vi "1-Main Image segmentation.vi"() -> ()   [LabVIEW 2015]
uses:
  <vilib>/Utility/file.llb/Read Delimited Spreadsheet (string).vi
  Dll/HyperImageBinarization.dll
panel:
  out "Image":T1(plugin-control)
  in  "secondOTSUMultiple":dbl
  in  "firstOTSUMultiple":dbl=0.94
  out "Current process of inter cycles":i32
  out "Number of inter cycles":i32
  out "Current process of external cycles":i32
  out "Number of external cycles":i32
  in  "divisor":i32=131
  in  "dividend":i32=109
  out "Current binary file path":path
  out "Files under current path":string[](array[string])
  out "lineNumbers":i32=340
  in  "waveSamples":i32=1004
  in  "waveNumbers":i32=250
  out "path":path
  in  "Binary path":path=path "I:/2017 Maize-Hyper-Program/2017 Maize Test sample/path.txt"
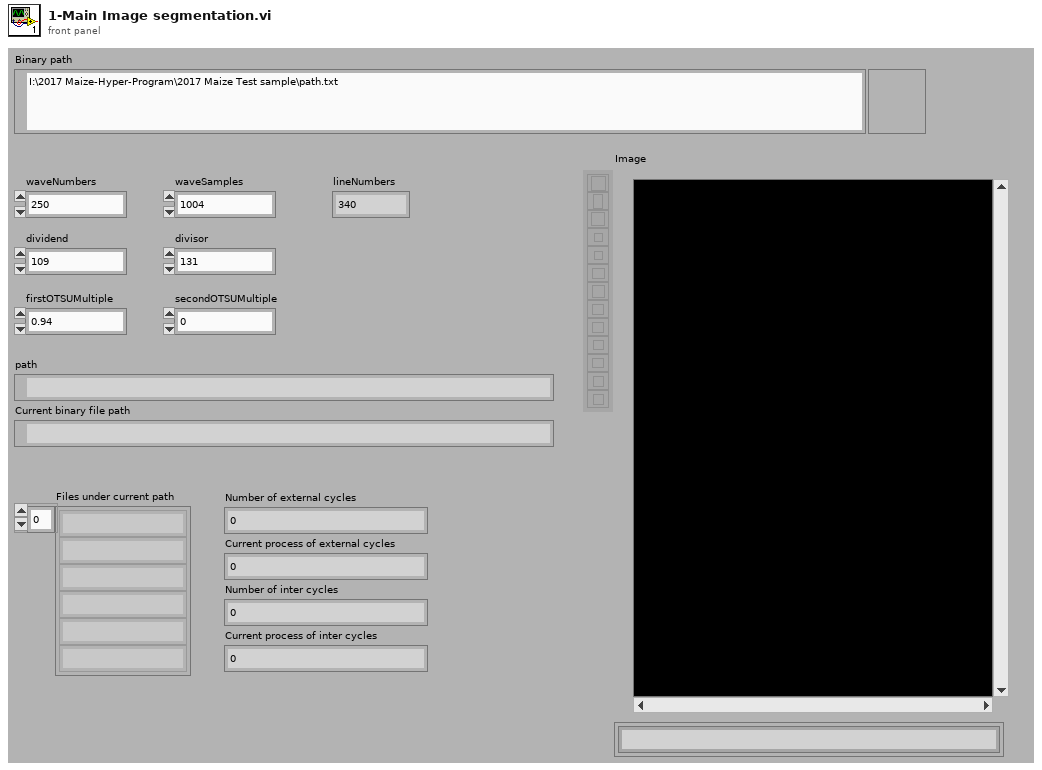
[diagram p1: front panel]
types:
  T1 = typedef "IMAQ Image.ctl" = refnum<image>
  T2 = typedef "Image Type" = u32
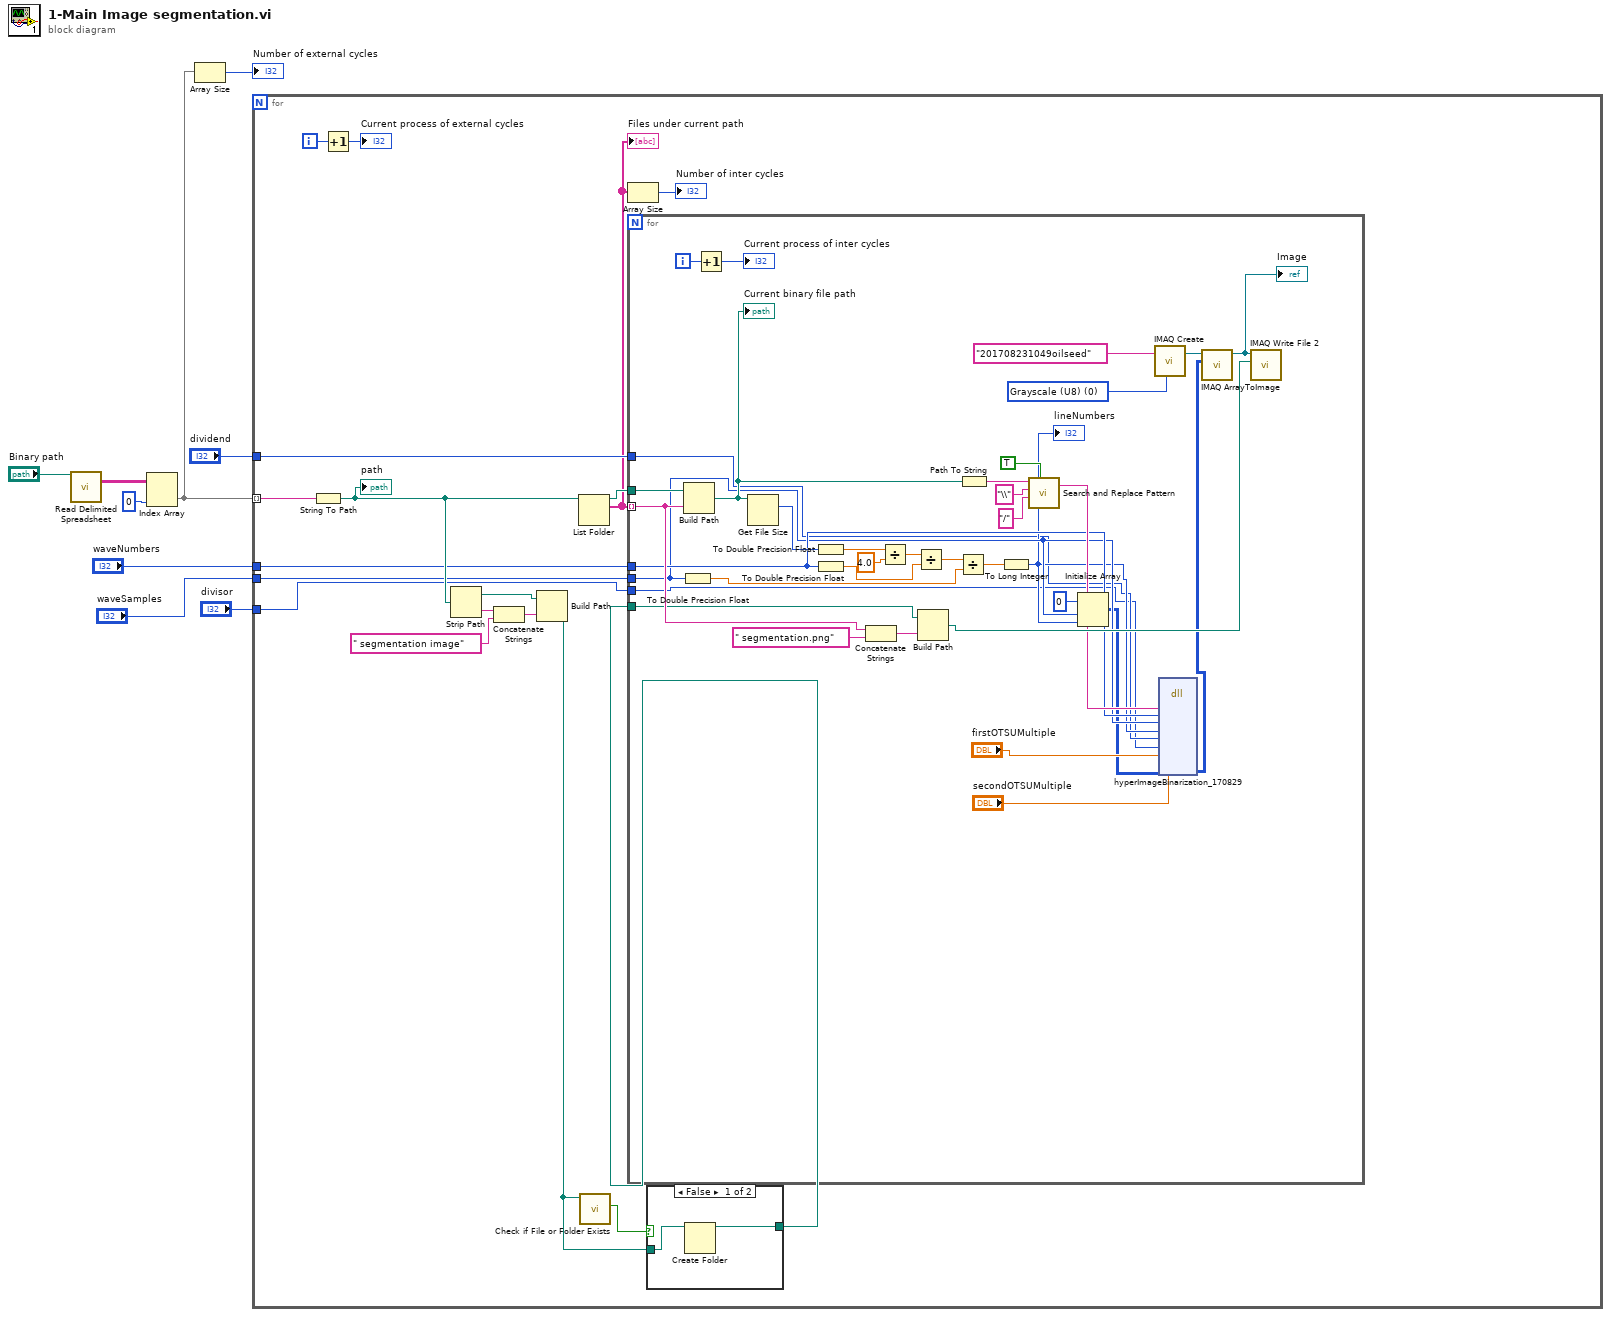
[diagram p0: block diagram]
diagram:
  n1 = call-poly <vilib>:"Read Delimited Spreadsheet.vi"("file path (dialog if empty)"="Binary path") -> ("all rows"=w5:string[][])  [unwired: 9 in, 5 out]
  n2 = Index Array(array=w5, index (col)=0 ("disabled index (col)")) -> (element=w2:string[])  [unwired: 1 in]
  n3 = Array Size(array=w2) -> (size(s)=→"Number of external cycles":i32)
  n4 = for {
    tunnel: w2 -> [w27] mode=indexing
    tunnel: "waveNumbers" -> [w20]
    tunnel: "waveSamples" -> [w19]
    tunnel: "dividend" -> [w18]
    tunnel: "divisor" -> [w17]
    i -> [w14]
    n5 = String To Path(string=w27) -> (path=w25:path)
    "path" <- w25
    n6 = Increment(x=w14) -> (x+1=→"Current process of external cycles":i32)
    n7 = Strip Path(path=w25) -> (stripped path=w22:path, name=w24:string)
    n8 = Concatenate Strings(w24, " segmentation image" ("string")) -> (w21:string)
    n9 = Build Path(base path=w22, name or relative path=w21) -> (appended path=w11:path)
    n10 = List Folder(path=w25) -> (path out=w26:path, filenames=w16:string[])  [unwired: 1 in, 4 out]
    "Files under current path" <- w16
    n11 = call <vilib>:"Check if File or Folder Exists.vi"("path"=w11) -> ("file or folder exists?"=w10:bool)  [unwired: 8 in, 2 out]
    n12 = Array Size(array=w16) -> (size(s)=→"Number of inter cycles":i32)
    n13 = case shown="False" w10 {
      tunnel: w11 -> [w29 w30]
      tunnel: [w28 w30] -> w12
      frame False {
        n14 = Create Folder(path (use dialog)=w29) -> (created path=w28:path)  [unwired: 1 in, 3 out]
      }
      frame True {
      }
    }
    n15 = for {
      tunnel: w26 -> [w66]
      tunnel: w16 -> [w61] mode=indexing
      tunnel: w12 -> [w59]
      tunnel: w20 -> [w40]
      tunnel: w19 -> [w39]
      tunnel: w18 -> [w37]
      tunnel: w17 -> [w36]
      i -> [w52]
      w54 = T2 0 items=["Grayscale (U8)", "Grayscale (I16)", "Grayscale (SGL)", "Complex (CSG)", "RGB (U32)", "HSL (U32)", "RGB (U64)", "Grayscale (U16)"] ("Image Type")
      n16 = To Double Precision Float(number=w39) -> (double precision float=w43:dbl)
      n17 = Build Path(base path=w66, name or relative path=w61) -> (appended path=w47:path)
      "Current binary file path" <- w47
      n18 = Increment(x=w52) -> (x+1=→"Current process of inter cycles":i32)
      n19 = Get File Size(file=w47) -> (size (in bytes)=w49:i64)  [unwired: 1 in, 2 out]
      n20 = To Double Precision Float(number=w49) -> (double precision float=w50:dbl)
      n21 = To Double Precision Float(number=w40) -> (double precision float=w45:dbl)
      n22 = Concatenate Strings(w61, " segmentation.png" ("string")) -> (w58:string)
      n23 = Divide(x=w50, y=4.0) -> (x/y=w46:dbl)
      n24 = Divide(x=w46, y=w45) -> (x/y=w44:dbl)
      n25 = Build Path(base path=w59, name or relative path=w58) -> (appended path=w57:path)
      n26 = Divide(x=w44, y=w43) -> (x/y=w42:dbl)
      n27 = Path To String(path=w47) -> (string=w62:string)
      n28 = To Long Integer(number=w42) -> (32bit integer=w38:i32)
      "lineNumbers" <- w38
      n29 = call <vilib>:"Search and Replace Pattern.vi"("string"=w62, "regular expression (\"\")"="\\" ("regular expression (\"\")"), "replace string (\"\")"="/" ("replace string (\"\")"), "replace all? (F)"=TRUE) -> ("result string"=w41:string)  [unwired: 2 out]
      n30 = Initialize Array(u8 0 ("element"), w39, w38) -> (w33:u8[][])
      n31 = call "IMAQ Create"("Image Name"="201708231049oilseed", "Image Type"=w54) -> ("New Image"=w56:T1)  [unwired: 2 in, 2 out]
      n32 = dll-call lib="I:/2017 Maize-Hyper-Program/Dll/HyperImageBinarization.dll" fn="hyperImageBinarization_170829"("filename"=w41, "wavenumbers"=w40, "wavesamples"=w39, "linenumbers"=w38, "dividend"=w37, "divisor"=w36, "firstOTSUMultiple"="firstOTSUMultiple", "secondOTSUMultiple"="secondOTSUMultiple", "output"=w33) -> ("output"=w32:u8[][])  [unwired: 11 in, 3 out]
      n33 = call "IMAQ ArrayToImage"("Image Pixels (U8)"=w32, "Image"=w56) -> ("Image Out"=w31:T1)  [unwired: 4 in, 5 out]
      "Image" <- w31
      n34 = call-poly "IMAQ Write File 2"("File Path"=w57, "Image"=w31) -> ()  [unwired: 4 in, 6 out]
    }
  }
